vi "Client Dashboard PC 1.vi"() -> ()   [LabVIEW 2016]
uses:
  <vilib>/Rock Robotics/Network Tables/NT Read String.vi
  <vilib>/Rock Robotics/Network Tables/NT Read Number.vi
panel:
  out "PDP Currents":T1
  out "Hopper Calculated Angle":dbl
  out "Hopper POT":dbl
  in  "stop":bool
  out "NAV X Readings":T2 {"Yaw" scale=0.0..360.0}
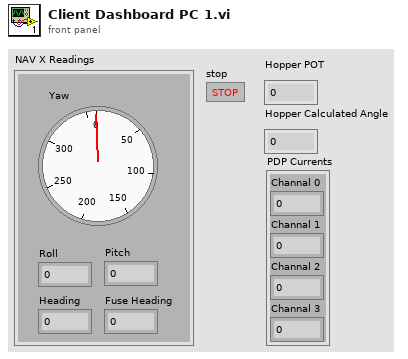
[diagram p1: front panel]
types:
  T1 = cluster{"Channal 0":dbl, "Channal 1":dbl, "Channal 2":dbl, "Channal 3":dbl}
  T2 = cluster{"Yaw":dbl, "Roll":dbl, "Pitch":dbl, "Heading":dbl, "Fuse Heading":dbl}
  T3 = cluster{"Numeric":dbl, "Numeric":dbl, "Numeric":dbl, "Numeric":dbl}
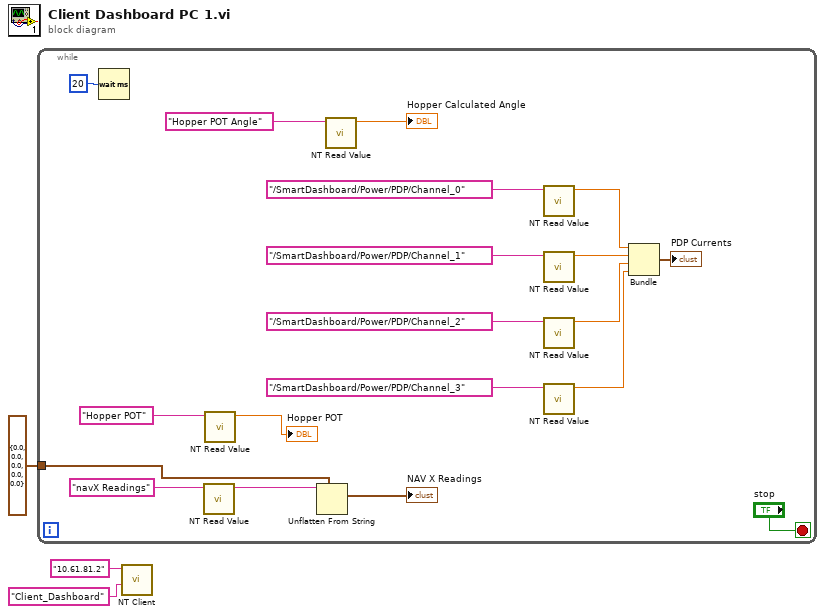
[diagram p0: block diagram]
diagram:
  n1 = while {
    tunnel: T2 {"Yaw"=0.0, "Roll"=0.0, "Pitch"=0.0, "Heading"=0.0, "Fuse Heading"=0.0} ("NAV X Readings") -> [w19]
    stop <- "stop" stop-if-true
    n2 = Wait (ms)(milliseconds to wait=u32 20) -> ()  [unwired: 1 out]
    n3 = call-poly <vilib>:"NT Read Value.vi"("Name"="navX Readings") -> ("String"=w20:string)  [unwired: 9 in, 1 out]
    n4 = call-poly <vilib>:"NT Read Value.vi"("Name"="Hopper POT") -> ("Numeric"=→"Hopper POT":dbl)  [unwired: 9 in, 1 out]
    n5 = Unflatten From String(type=w19, binary string=w20) -> (value=→"NAV X Readings":T2)  [unwired: 3 in, 2 out]
    n6 = call-poly <vilib>:"NT Read Value.vi"("Name"="Hopper POT Angle") -> ("Numeric"=→"Hopper Calculated Angle":dbl)  [unwired: 9 in, 1 out]
    n7 = call-poly <vilib>:"NT Read Value.vi"("Name"="/SmartDashboard/Power/PDP/Channel_0") -> ("Numeric"=w9:dbl)  [unwired: 9 in, 1 out]
    n8 = call-poly <vilib>:"NT Read Value.vi"("Name"="/SmartDashboard/Power/PDP/Channel_1") -> ("Numeric"=w8:dbl)  [unwired: 9 in, 1 out]
    n9 = call-poly <vilib>:"NT Read Value.vi"("Name"="/SmartDashboard/Power/PDP/Channel_2") -> ("Numeric"=w7:dbl)  [unwired: 9 in, 1 out]
    n10 = call-poly <vilib>:"NT Read Value.vi"("Name"="/SmartDashboard/Power/PDP/Channel_3") -> ("Numeric"=w6:dbl)  [unwired: 9 in, 1 out]
    n11 = Bundle("Numeric"=w9, "Numeric"=w8, "Numeric"=w7, "Numeric"=w6) -> (→"PDP Currents":T3)  [unwired: 1 in]
  }
  n12 = call <vilib>:"NT Client.vi"("Client Name"="Client_Dashboard", "Server IP Address"="10.61.81.2") -> ()  [unwired: 10 in]
